vi "TLPM Close2.vi"(8 "error in (no error)":errorcluster, 11 "instrument handle":refnum<visa-resource-name>) -> (0 "error out":errorcluster)   [LabVIEW 2018, in "Power Meter.lvlib"]
doc: "This VI closes the instrument driver session.\n\nNote: The instrument must be reinitialized to use it again."
uses:
  Power Meter.lvlib
  TLPM_64.dll
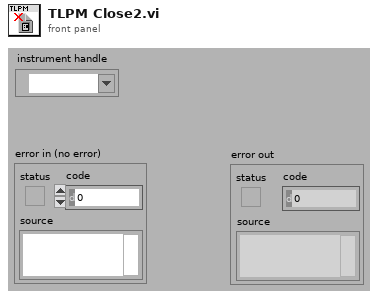
[diagram p1: front panel]
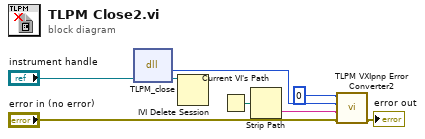
[diagram p0: block diagram]
diagram:
  n1 = dll-call lib="TLPM_64.dll" fn="TLPM_close"("instrument handle"="instrument handle") -> ("status"=w2:i32)  [unwired: 4 in, 2 out]
  n2 = IVI Delete Session(11:"instrument handle") -> ()
  n3 = Current VI's Path() -> (path=w7:path)
  n4 = Strip Path(path=w7) -> (name=w3:string)  [unwired: 1 out]
  n5 = call "TLPM VXIpnp Error Converter2.vi"("error in (no error)"="error in (no error)", "Name Of VI (\"\")"=w3, "CVI Error Code (0)"=w2, "instrument handle"=i8 0) -> ("error out"=→"error out":errorcluster)  [unwired: 6 in, 1 out]
